vi "SetLightTower&Switch.vi"(6 "Supress Match Error (F)":bool, 8 "error in (no error)":errorcluster, 9 "UpdateValue? (F)":bool[](array[boolean]), 10 "RoomAlert Device":T1, 11 "RoomAlert in":refnum<class "RoomAlert.lvclass">) -> (0 "error out":errorcluster, 3 "RoomAlert out":refnum<class "RoomAlert.lvclass">)   [LabVIEW 2018, in "SensorPlugins.lvlib" / "RoomAlert.lvclass"]
doc: "Sets the LED and audio value of the LightTower alarm."
uses:
  RoomAlert.lvclass
  TypeDefinitions/RoomAlertControls.ctl
  RoomAlert.lvclass/RoomAlert.ctl
  <vilib>/Utility/error.llb/Error Cluster From Error Code.vi
  <vilib>/ErrorRing/Error Ring.xnode
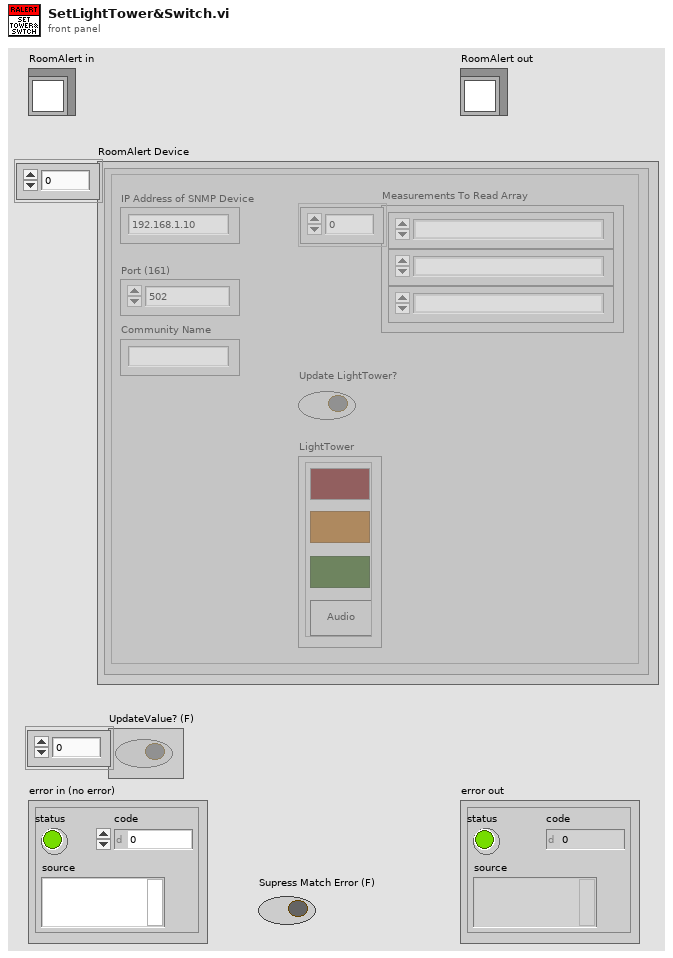
[diagram p1: front panel]
types:
  T1 = typedef "SensorPlugins.lvlib/RoomAlert.lvclass/RoomAlertControls.ctl" = cluster{"Connected?":bool, "IP Address of SNMP Device":string, "Port (161)":u16, "Community Name":string, "Measurements To Read Array":u16[], "Update LightTower?":bool, "LightTower":cluster{"Red":bool, "Amber":bool, "Green":bool, "Audio":bool}}[]
  T2 = typedef "SensorPlugins.lvlib/RoomAlert.lvclass/ValuesToSet.ctl" = string[][][]
  T3 = typedef "SensorPlugins.lvlib/RoomAlert.lvclass/MeasurementControls.ctl" = cluster{"Measurement RefreshTime (ms)":u32, "Measurement Name":string, "Timeout(ms)":i32, "Amber Warning Light Configuration":cluster{"Warning Temperture (Degrees C)":dbl, "Temperature Delta (Degrees C/Minute)":dbl, "Time Window (Minutes)":dbl}}
  T4 = cluster{"Red":bool, "Amber":bool, "Green":bool, "Audio":bool}
  T5 = typedef "SensorPlugins.lvlib/RoomAlert.lvclass/CommunicationControls.ctl" = refnum<k16>[]
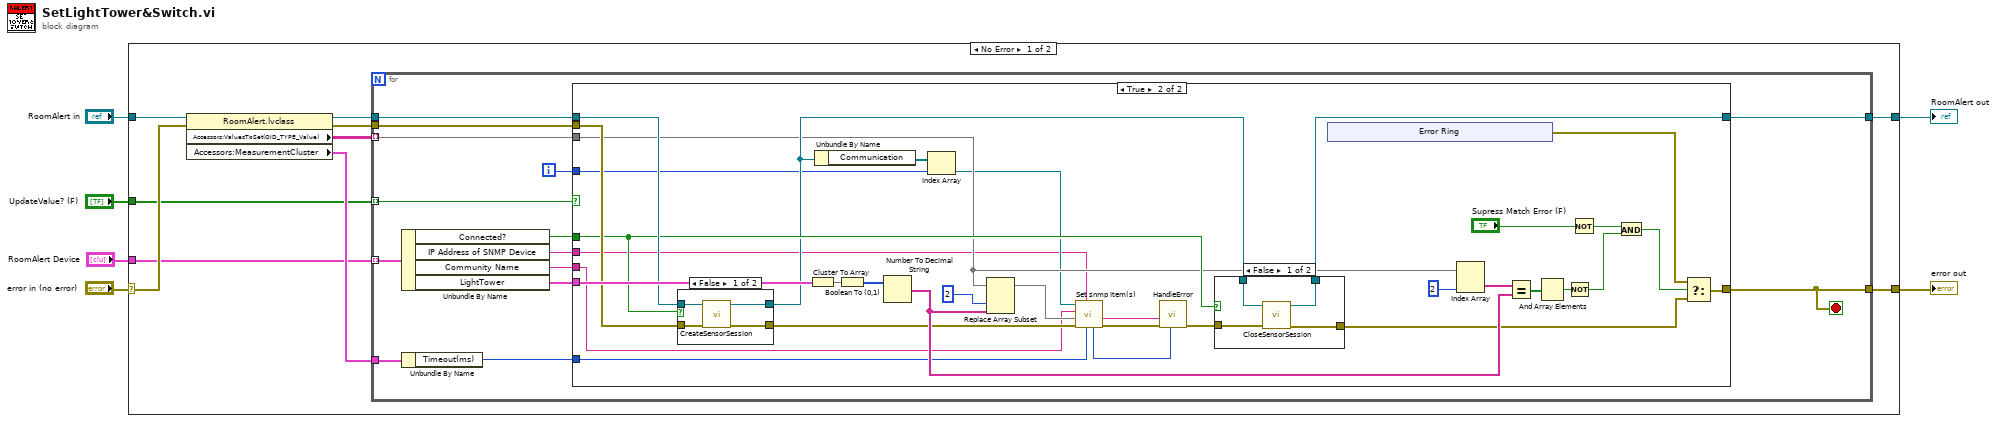
[diagram p0: block diagram]
diagram:
  n1 = case shown="No Error" "error in (no error)" {
    selector: "error in (no error)" -> [w15 w85]
    tunnel: [w13 w85] -> w5
    tunnel: [w11 w84] -> w3
    tunnel: "RoomAlert in" -> [w16 w84]
    tunnel: "RoomAlert Device" -> [w8 _]
    tunnel: "UpdateValue? (F)" -> [w7 _]
    frame No Error {
      n2 = property class="RoomAlert.lvclass"(reference=w16, error in=w15) -> (reference out=w12:refnum<class "RoomAlert.lvclass">, error out=w14:errorcluster, "Accessors:ValuesToSet(OID_TYPE_Value)"=w9:T2, "Accessors:MeasurementCluster"=w10:T3)
      n3 = for {
        tunnel: w8 -> [w30] mode=indexing
        tunnel: w14 -> [w20]
        tunnel: [w26] -> w13
        tunnel: w12 -> [w23]
        tunnel: [w22] -> w11
        tunnel: w10 -> [w25]
        tunnel: w9 -> [w21] mode=indexing
        tunnel: w7 -> [w18] mode=indexing
        i -> [w17]
        stop <- w26 stop-if-true
        n4 = Unbundle By Name(w30) -> ("Connected?"=w19:bool, "IP Address of SNMP Device"=w27:string, "Community Name"=w28:string, "LightTower"=w29:T4)
        n5 = Unbundle By Name(w25) -> ("Timeout(ms)"=w24:i32)
        n6 = case shown="True" w18 {
          tunnel: w29 -> [_ w66]
          tunnel: w28 -> [_ w37]
          tunnel: w27 -> [_ w38]
          tunnel: w21 -> [_ w46]
          tunnel: [w31 w65] -> w26
          tunnel: w24 -> [_ w42]
          tunnel: w23 -> [w32 w51]
          tunnel: [w32 w53] -> w22
          tunnel: w20 -> [w31 w52]
          tunnel: w19 -> [_ w50]
          tunnel: w17 -> [_ w47]
          frame False {
          }
          frame True {
            n7 = case shown="False" w50 {
              tunnel: w52 -> [w70 w72]
              tunnel: [w69 w72] -> w45
              tunnel: w51 -> [w68 w71]
              tunnel: [w67 w71] -> w49
              frame False {
                n8 = call-dynamic "CreateSensorSession.vi"("error in (no error)"=w70, "RoomAlert in"=w68) -> ("error out"=w69:errorcluster, "RoomAlert out"=w67:refnum<class "RoomAlert.lvclass">)  [unwired: 8 in]
              }
              frame True {
              }
            }
            n9 = Cluster To Array(cluster=w66) -> (array=w64:bool[])
            n10 = Unbundle By Name(w49) -> ("Communication"=w48:T5)
            n11 = Boolean To (0,1)(Boolean=w64) -> (0, 1=w63:i16[])
            n12 = Number To Decimal String(number=w63) -> (decimal integer string=w61:string[])  [unwired: 1 in]
            n13 = Index Array(array=w48, index=w47) -> (element=w40:refnum<k16>)
            n14 = Replace Array Subset(array=w46, new element=w61, index (col)=2 ("disabled index (col)")) -> (w39:string[][])  [unwired: 1 in]
            n15 = call "Set snmp Item(s).vi"("timeout ms (25000)"=w42, "IP Address of SNMP Device"=w38, "error in (no error)"=w45, "OID/TYPE/VALUE ARRAY"=w39, "Community Name"=w37, "connection ID in"=w40) -> ("error out"=w44:errorcluster, "error-string"=w43:string, "error-status"=w41:u8)  [unwired: 3 out]
            n16 = call "HandleError.vi"("error-status"=w41, "Error In"=w44, "Error String"=w43) -> ("Error Out"=w55:errorcluster)  [unwired: 8 in]
            n17 = case shown="False" w50 {
              tunnel: w55 -> [w76 w77]
              tunnel: [w75 w77] -> w54
              tunnel: [w74 w78] -> w53
              tunnel: w49 -> [w73 w78]
              frame False {
                n18 = call-dynamic "CloseSensorSession.vi"("error in (no error)"=w76, "RoomAlert in"=w73) -> ("error out"=w75:errorcluster, "RoomAlert out"=w74:refnum<class "RoomAlert.lvclass">)  [unwired: 8 in]
              }
              frame True {
              }
            }
            n19 = xnode "Error Ring"() -> ("error out"=w56:errorcluster)
            n20 = Index Array(array=w46, index (col)=2 ("disabled index (col)")) -> (element=w59:string[])  [unwired: 1 in]
            n21 = Equal?(x=w59, y=w61) -> (x = y?=w58:bool[])
            n22 = And Array Elements(Boolean array=w58) -> (logical AND=w57:bool)
            n23 = Not(x=w57) -> (.not. x?=w34:bool)
            n24 = Not(x="Supress Match Error (F)") -> (.not. x?=w35:bool)
            n25 = And(x=w35, y=w34) -> (x .and. y?=w33:bool)
            n26 = Select(t=w56, s=w33, f=w54) -> (s? t:f=w65:errorcluster)
          }
        }
      }
    }
    frame Error {
    }
  }
  "error out" <- w5
  "RoomAlert out" <- w3
